vi "Alarms Wizard.vi"(8 "error in":errorcluster, 11 "Shared Variable Name":string) -> (0 "error out":errorcluster, 2 "Cancel":bool, 3 "alarm settings":T1={"enable? (F)"=FALSE, "name"="HiHi", "alarm type"=enum."HI_HI", "level/change"=90.0, "deadband/time"=1.0, "priority"=1, "ack type"=enum."Auto", "area"="", "description"="", "log? (T)"=TRUE} {"priority" min=1 max=5000})   [LabVIEW 2020]
uses:
  <vilib>/lvdsc/variables/internal/AlarmSettings_Numeric.ctl
  <vilib>/lvdsc/variables/internal/NumericAlarmType.ctl
panel:
  in  "OK Button":bool
  in  "Cancel Button":bool
  in  "Next Button":bool
  in  "Previous Button":bool
  in  "Tab Control":enum32{"1", "2", "3", "4", "5", "6", "7"}(tab)
  in  "alarm type":enum16{"HI_HI", "HI", "LO", "LO_LO"}(ring)
  in  "Set Point":dbl
  in  "deadband":dbl
  in  "priority":enum16{"Low", "Moderate", "High", "Critical"}(ring)
  in  "area":string
  in  "description":string
  in  "log?":bool
  # "Select the Alarm Type"
  # "Users may configure upto 4 alarms for each\nvariable. \nHI_HI and HI are High level Alarms\ntriggered when varaible value goes over the\nsetpoint. \nLO_LO and LO are Low level alarms\nthat are triggered when variable value falls\nbelow the setpoint."
  # "Enter the Set Point"
  # "A setpoint is the threshold for the alarm. The \nalarm is trigger when variable value crosses\nthis threshold."
  # "Enter the deadband"
  # "Deadband is range of values above or below \nthe alarm threshold. It prevents frequent\ntoggling of alarms if the variable value is \nnoisy around the threshold value.\n\nFor example, if the Setpoint for a HI alarm is \n1200 and the deadband is 50, the alarm will be \ntriggered when the variable value is greater\nthan 1200 and will remain Active until it falls\nbelow 1150."
  # "Set the Priority Level"
  # "The Priority Level allows the user to set up \nthe severity of the alarm. There are 4 levels\navailable. User alerts for alarms vary based on\nthe priority level set for the alarm."
  # "Enter Area/Location"
  # "Provide the name of the Area for which the \nvaraible is being logged and monitored\nfor alarms."
  # "Enter Description"
  # "Provide a description for the Alarm. \nFor example, \" Hi Alarm for Cryo1 Temp\""
  # "Do you want to Log this Alarm?"
  # "Click on this button to toggle between choices.\nUsers may choose to log this alarm event\nin a database. This will provide a history for\nthis alarm."
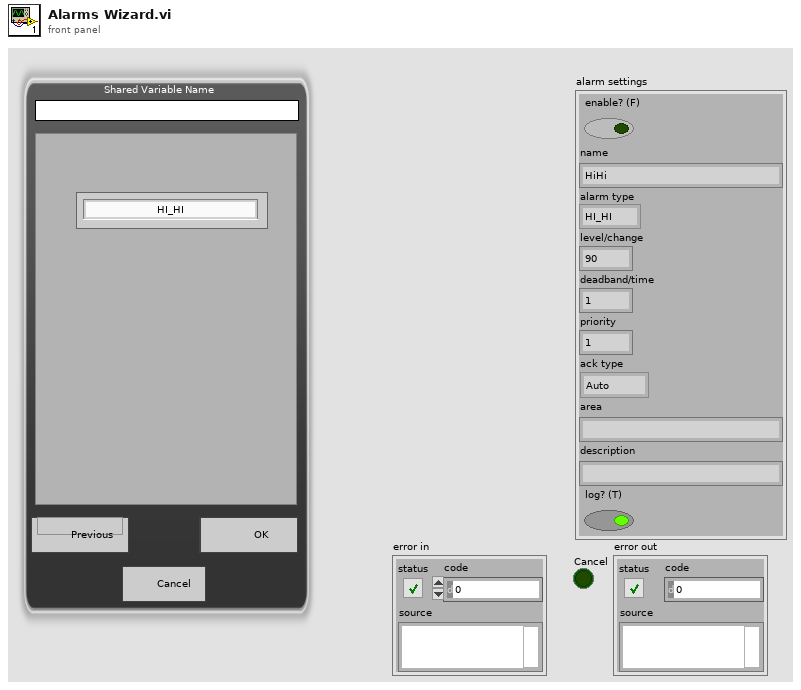
[diagram p1: front panel]
types:
  T1 = typedef "AlarmSettings_Numeric.ctl" = cluster{"enable? (F)":bool, "name":string, "alarm type":T2, "level/change":dbl, "deadband/time":dbl, "priority":u32, "ack type":enum16{"Auto", "User", "None", "Each Occurrence"}, "area":string, "description":string, "log? (T)":bool}
  T2 = typedef "NumericAlarmType.ctl" = enum16{"HI_HI", "HI", "LO", "LO_LO"}
  T3 = enum32{"invalid app kind", "Development System", "Run Time System", "Student Edition", "Embedded LabVIEW", "Evaluation", "Custom"}
  T4 = enum32{"Invalid", "Standard", "Closed", "Hidden", "Minimized", "Maximized"}
  T5 = cluster{"Core":cluster{"Current VI Reference":refnum<vi>, "Close Panel on Exit?":bool}, "No of pages":i32, "alarm settings":T1}
  T6 = cluster{"Current VI Reference":refnum<vi>, "Close Panel on Exit?":bool}
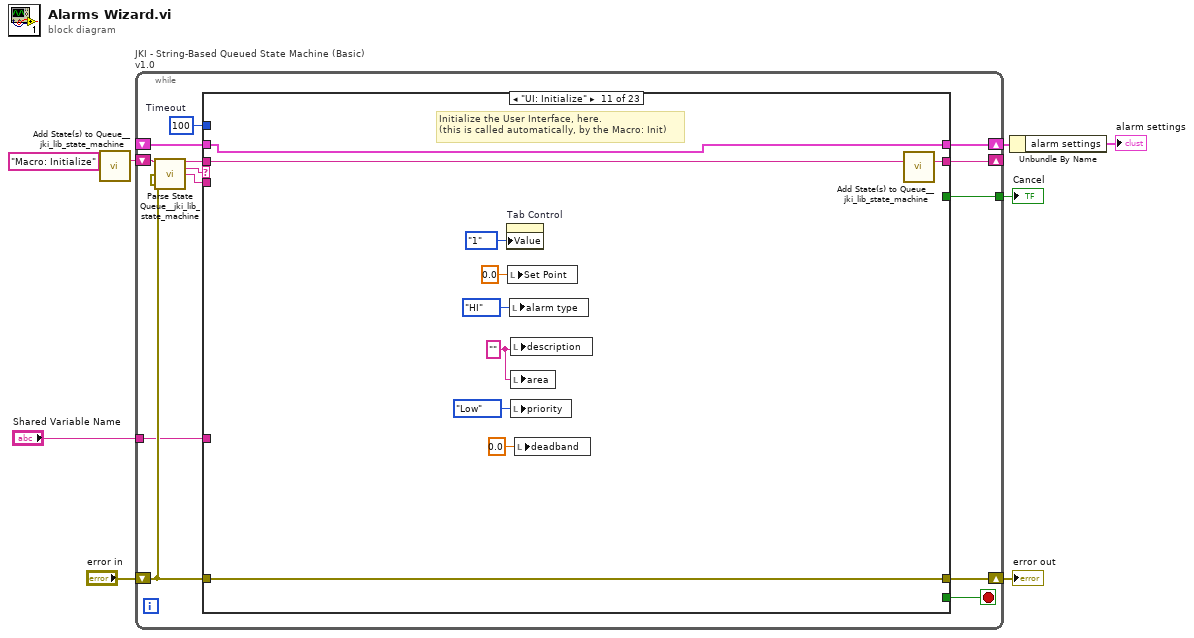
[diagram p0: block diagram]
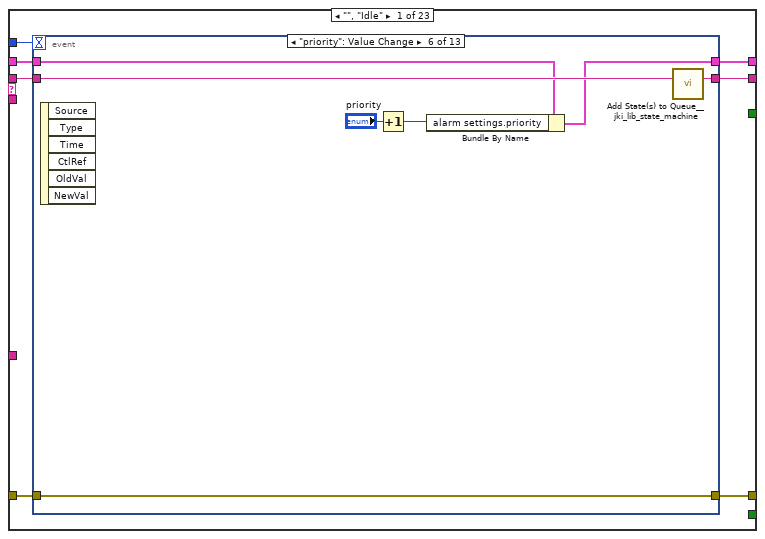
[diagram p2: hidden frame]
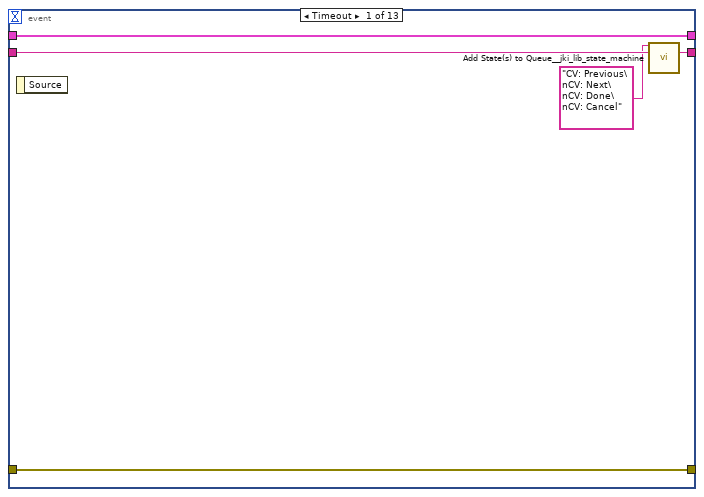
[diagram p3: hidden frame]
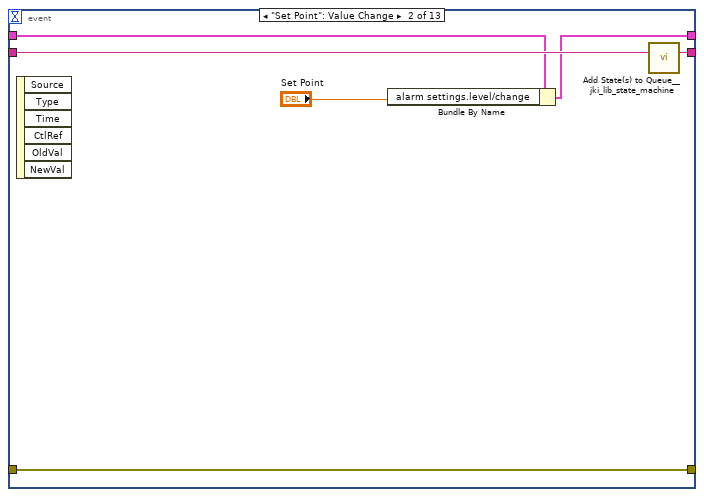
[diagram p4: hidden frame]
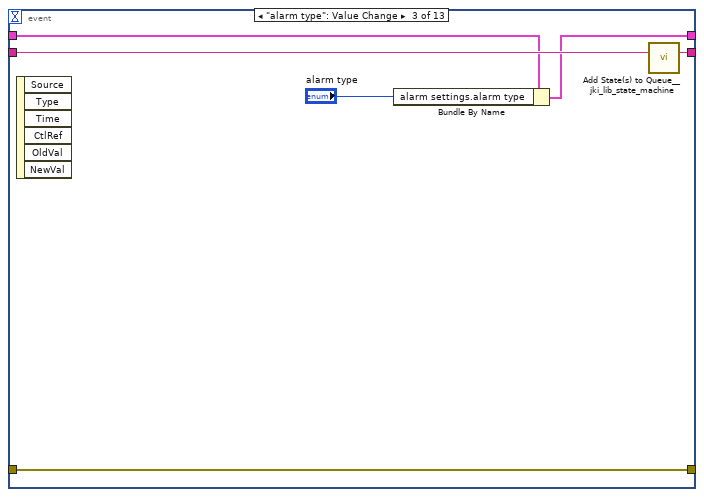
[diagram p5: hidden frame]
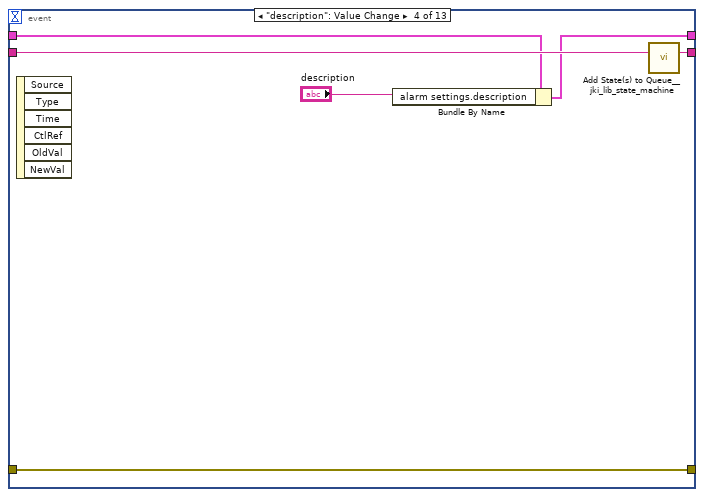
[diagram p6: hidden frame]
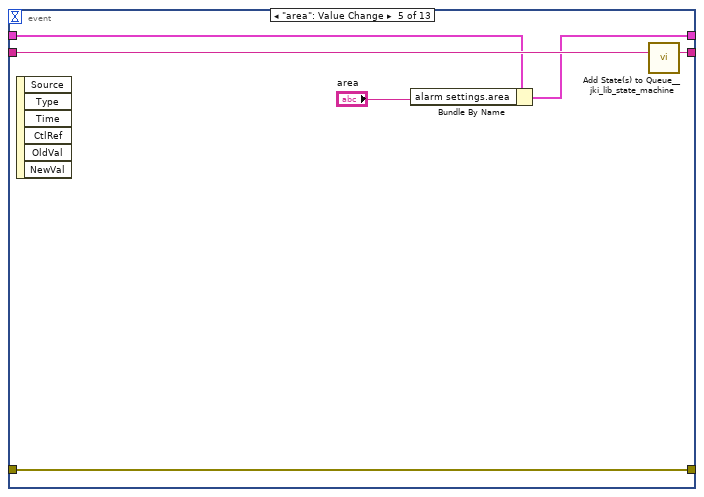
[diagram p7: hidden frame]
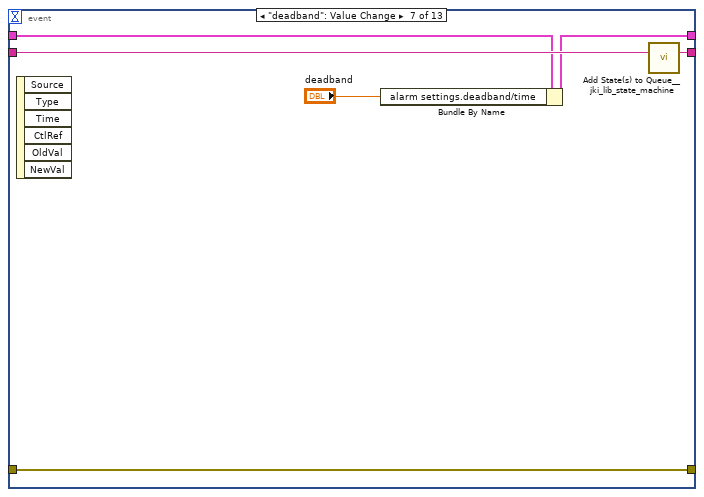
[diagram p8: hidden frame]
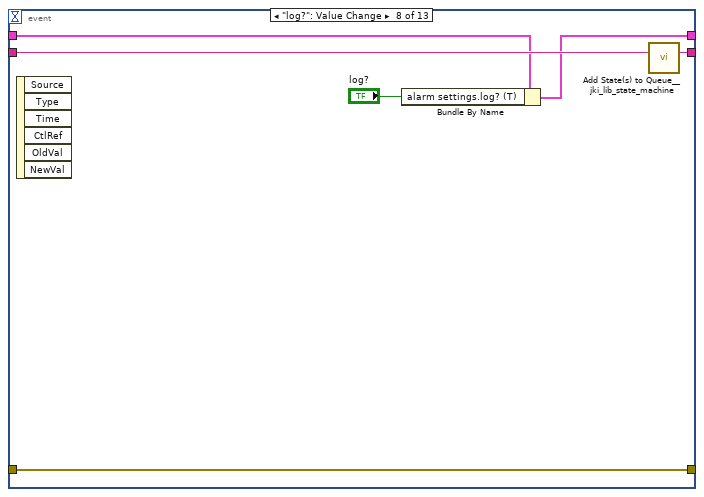
[diagram p9: hidden frame]
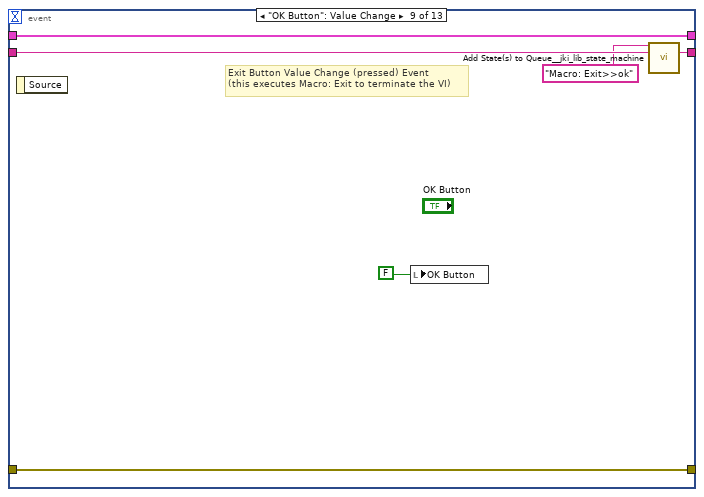
[diagram p10: hidden frame]
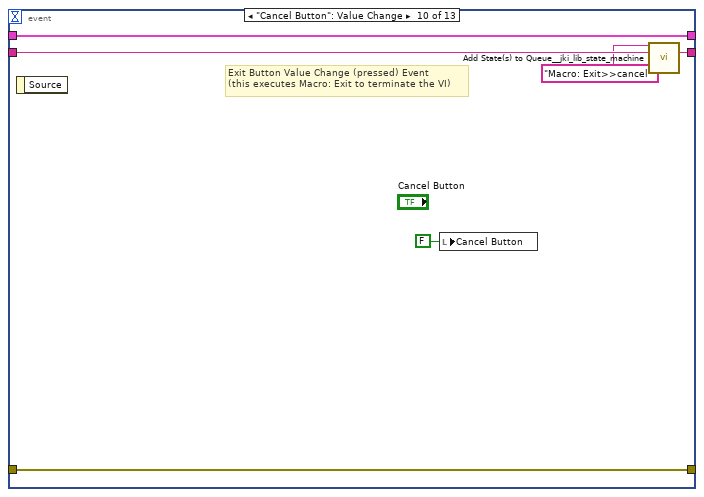
[diagram p11: hidden frame]
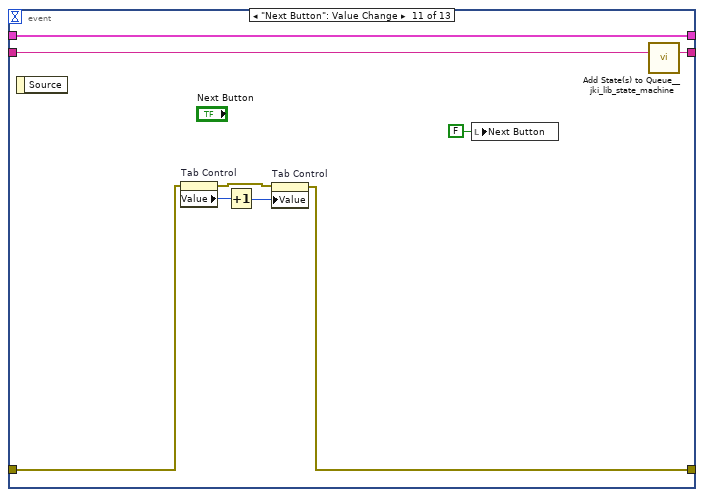
[diagram p12: hidden frame]
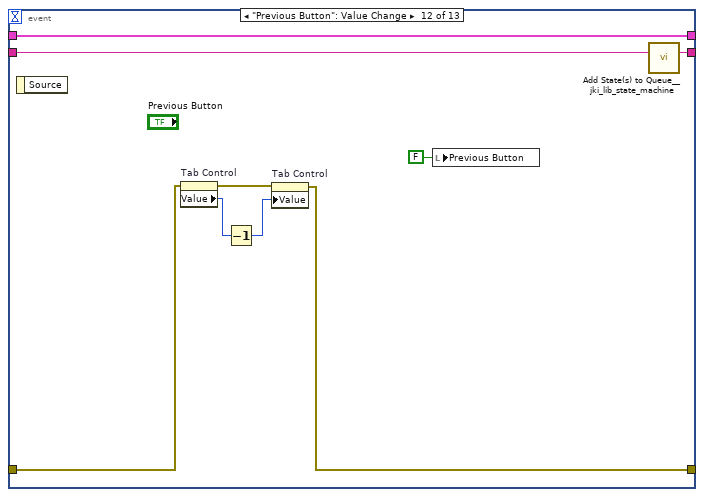
[diagram p13: hidden frame]
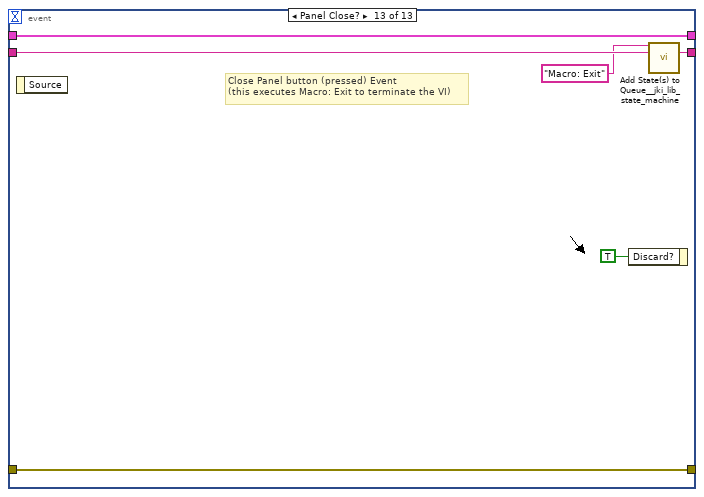
[diagram p14: hidden frame]
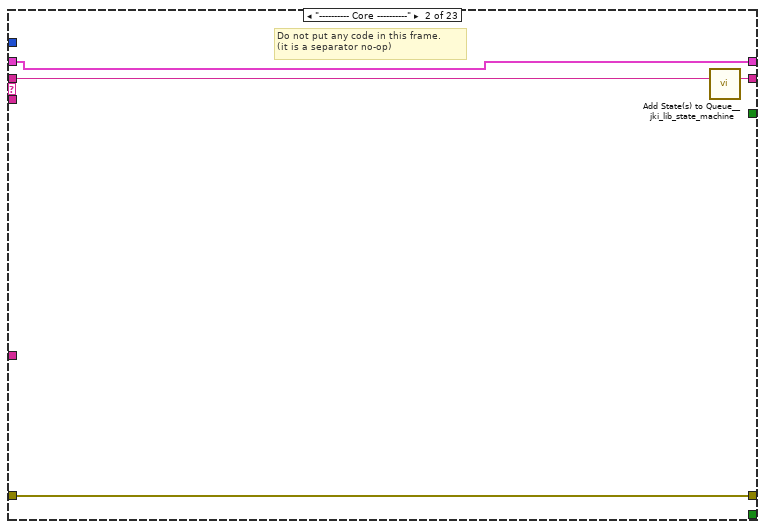
[diagram p15: hidden frame]
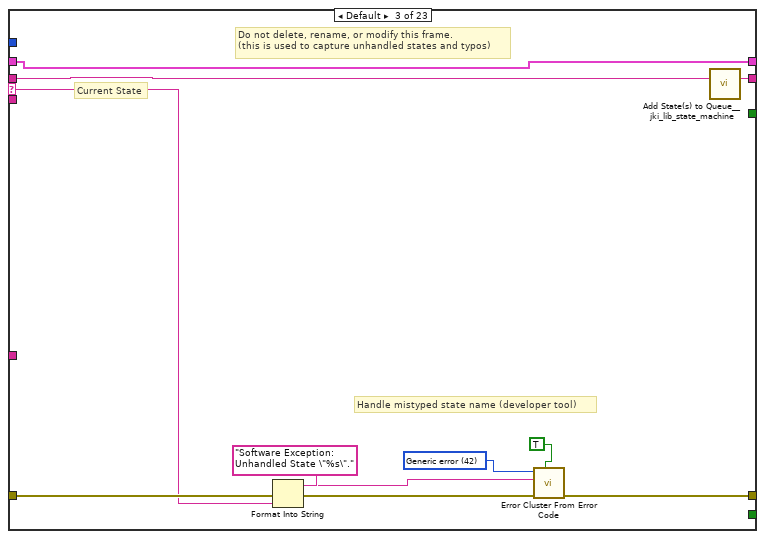
[diagram p16: hidden frame]
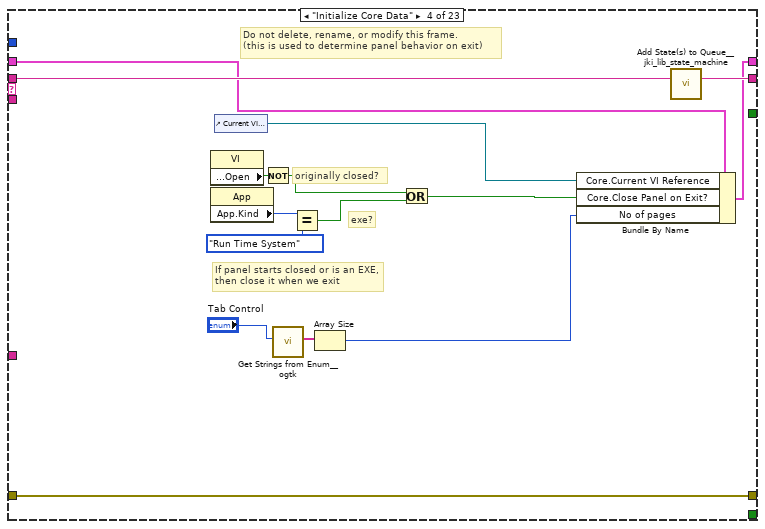
[diagram p17: hidden frame]
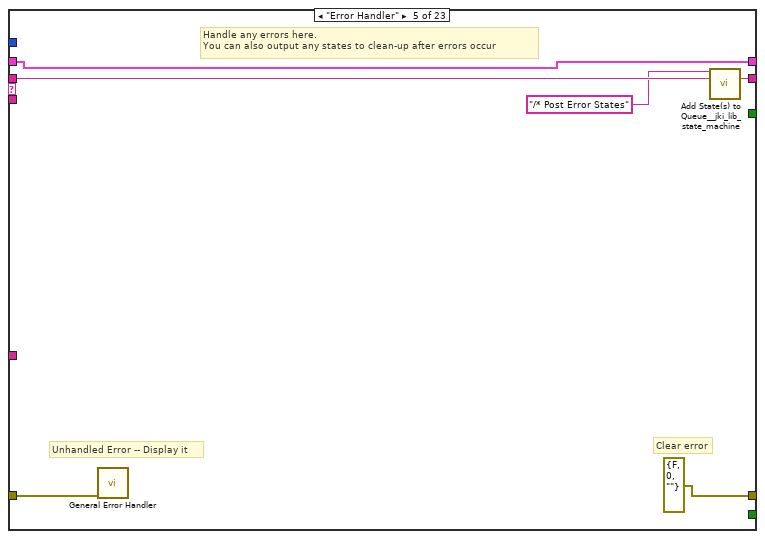
[diagram p18: hidden frame]
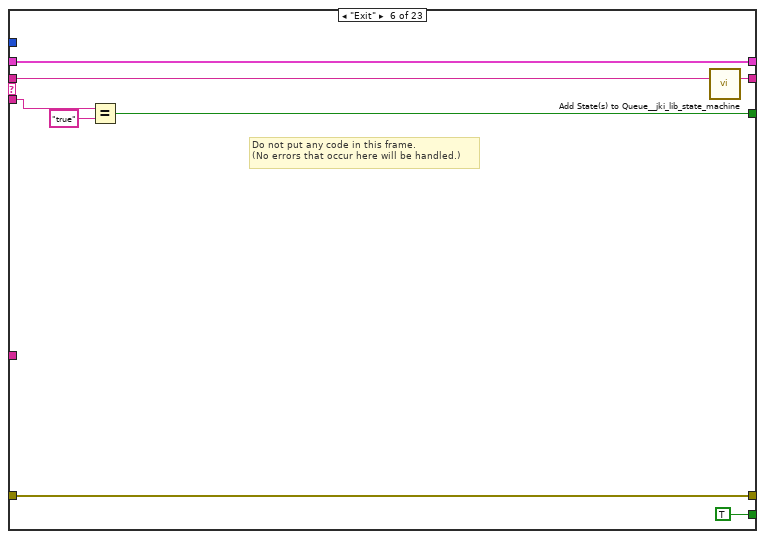
[diagram p19: hidden frame]
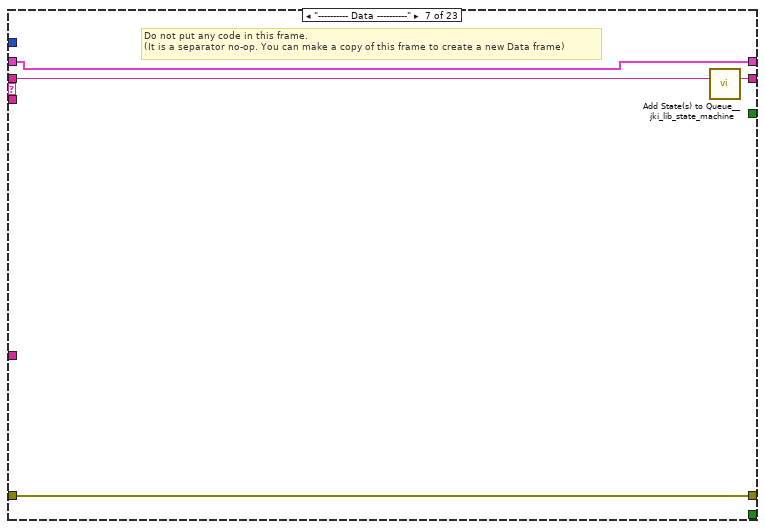
[diagram p20: hidden frame]
diagram:
  n1 = call <vilib>:"Add State(s) to Queue__jki_lib_state_machine.vi"("State(s) in (\"\")"="Macro: Initialize") -> ("States Out"=w8:string)  [unwired: 14 in]
  n2 = while "JKI - String-Based Queued State Machine (Basic) v1.0" {
    shift-right: [w14] -> w4
    shift-left: _ -> [w13]
    shift-right: [w17] -> w1
    shift-left: "error in" -> [w11]
    shift-right: [w16] -> _
    shift-left: w8 -> [w18]
    tunnel: "Shared Variable Name" -> [w10]
    tunnel: [w9] -> w5
    stop <- w15 stop-if-true
    w12 = 100  # Timeout
    n3 = call <vilib>:"Parse State Queue__jki_lib_state_machine.vi"("State Queue"=w18, "Error In (no error)"=w11) -> ("Remaining States"=w20:string, "Current State"=w21:string, "Arguments"=w19:string)  [unwired: 11 in]
    n4 = case shown="\"UI: Initialize\"" w21 {
      selector: w21 -> [_ _ w117 _ _ _ _ _ _ _ _ _ _ _ _ _ _ _ _ _ _ _ _]
      tunnel: w20 -> [w28 w116 w121 w142 w148 w156 w160 w169 w175 w179 w189 w195 w206 w232 w237 w252 w256 w265 w276 w286 w290 w294 w298]
      tunnel: w19 -> [_ _ _ _ _ w151 _ _ _ _ _ w190 w200 _ _ w243 _ _ _ _ _ _ _]
      tunnel: w13 -> [w26 w113 w119 w133 w145 w154 w157 _ w170 w176 w187 w193 w202 w229 w234 w249 w253 w262 w273 w283 w287 w291 w295]
      tunnel: [w25 w114 w123 w139 errorcluster {"status"=FALSE, "code"=0, "source"=""} ("error out") w153 w158 w166 w171 w177 w186 w191 w203 w230 w235 w250 w254 w257 w274 w284 w288 w292 w296] -> w17
      tunnel: w11 -> [w24 w114 w122 w139 w144 w153 w158 w166 w172 w177 w186 w192 w204 w230 w235 w250 w254 w258 w274 w284 w288 w292 w296]
      tunnel: [w27 w115 w120 w141 w147 w155 w159 w168 w174 w178 w188 w194 w205 w231 w236 w251 w255 w264 w275 w285 w289 w293 w297] -> w16
      tunnel: [_ _ _ _ _ TRUE _ _ _ _ _ _ _ _ _ _ _ _ _ _ _ _ _] -> w15
      tunnel: [w23 w113 w119 w140 w145 w154 w157 w167 w170 w176 w187 w193 w202 w229 w234 w249 w253 w262 w273 w283 w287 w291 w295] -> w14
      tunnel: w12 -> [w22 _ _ _ _ _ _ _ _ _ _ _ _ _ _ _ _ _ _ _ _ _ _]
      tunnel: w10 -> [_ _ _ _ _ _ _ w162 _ _ _ _ _ _ _ _ _ _ _ _ _ _ _]
      tunnel: [_ _ _ _ _ w149 _ _ _ _ _ _ _ _ _ _ _ _ _ _ _ _ _] -> w9
      frame "", "Idle" {
        n5 = event shown="[5] \"priority\": Value Change" {
          selector: _ -> [_ _ _ _ _ _ _ _ _ _ _ _ _]
          dyn-events: _ -> [_ _ _ _ _ _ _ _ _ _ _ _ _]
          timeout: w22 -> [_ _ _ _ _ _ _ _ _ _ _ _ _]
          tunnel: w28 -> [w33 w39 w45 w51 w57 w64 w70 w76 w82 w88 w97 w106 w112]
          tunnel: [w32 w38 w44 w50 w56 w63 w69 w75 w81 w87 w96 w105 w111] -> w27
          tunnel: w26 -> [w30 w36 w42 w48 w54 w61 w67 w73 w79 w85 w95 w104 w109]
          tunnel: [w31 w37 w43 w49 w55 w62 w68 w74 w80 w86 w90 w99 w110] -> w25
          tunnel: w24 -> [w31 w37 w43 w49 w55 w62 w68 w74 w80 w86 w91 w100 w110]
          tunnel: [w30 w35 w41 w47 w53 w60 w66 w72 w79 w85 w95 w104 w109] -> w23
          event Timeout {
            n6 = event-data() -> ()  [unwired: 1 in, 1 out]
            n7 = call <vilib>:"Add State(s) to Queue__jki_lib_state_machine.vi"("State(s) in Front (\"\")"="CV: Previous\nCV: Next\nCV: Done\nCV: Cancel", "State(s) in (\"\")"=w33) -> ("States Out"=w32:string)  [unwired: 13 in]
          }
          event "Set Point": Value Change {
            n8 = event-data() -> ()  [unwired: 1 in, 6 out]
            n9 = Bundle By Name(cluster=w36, "alarm settings.level/change"="Set Point") -> (w35:T5)
            n10 = call <vilib>:"Add State(s) to Queue__jki_lib_state_machine.vi"("State(s) in (\"\")"=w39) -> ("States Out"=w38:string)  [unwired: 14 in]
          }
          event "alarm type": Value Change {
            n11 = event-data() -> ()  [unwired: 1 in, 6 out]
            n12 = Bundle By Name(cluster=w42, "alarm settings.alarm type"="alarm type") -> (w41:T5)
            n13 = call <vilib>:"Add State(s) to Queue__jki_lib_state_machine.vi"("State(s) in (\"\")"=w45) -> ("States Out"=w44:string)  [unwired: 14 in]
          }
          event "description": Value Change {
            n14 = event-data() -> ()  [unwired: 1 in, 6 out]
            n15 = Bundle By Name(cluster=w48, "alarm settings.description"="description") -> (w47:T5)
            n16 = call <vilib>:"Add State(s) to Queue__jki_lib_state_machine.vi"("State(s) in (\"\")"=w51) -> ("States Out"=w50:string)  [unwired: 14 in]
          }
          event "area": Value Change {
            n17 = event-data() -> ()  [unwired: 1 in, 6 out]
            n18 = Bundle By Name(cluster=w54, "alarm settings.area"="area") -> (w53:T5)
            n19 = call <vilib>:"Add State(s) to Queue__jki_lib_state_machine.vi"("State(s) in (\"\")"=w57) -> ("States Out"=w56:string)  [unwired: 14 in]
          }
          event "priority": Value Change {
            n20 = event-data() -> ()  [unwired: 1 in, 6 out]
            n21 = Increment(x="priority") -> (x+1=w58:enum16{"Low", "Moderate", "High", "Critical"})
            n22 = Bundle By Name(cluster=w61, "alarm settings.priority"=w58) -> (w60:T5)
            n23 = call <vilib>:"Add State(s) to Queue__jki_lib_state_machine.vi"("State(s) in (\"\")"=w64) -> ("States Out"=w63:string)  [unwired: 14 in]
          }
          event "deadband": Value Change {
            n24 = event-data() -> ()  [unwired: 1 in, 6 out]
            n25 = Bundle By Name(cluster=w67, "alarm settings.deadband/time"="deadband") -> (w66:T5)
            n26 = call <vilib>:"Add State(s) to Queue__jki_lib_state_machine.vi"("State(s) in (\"\")"=w70) -> ("States Out"=w69:string)  [unwired: 14 in]
          }
          event "log?": Value Change {
            n27 = event-data() -> ()  [unwired: 1 in, 6 out]
            n28 = Bundle By Name(cluster=w73, "alarm settings.log? (T)"="log?") -> (w72:T5)
            n29 = call <vilib>:"Add State(s) to Queue__jki_lib_state_machine.vi"("State(s) in (\"\")"=w76) -> ("States Out"=w75:string)  [unwired: 14 in]
          }
          event "OK Button": Value Change {
            # "Exit Button Value Change (pressed) Event\n(this executes Macro: Exit to terminate the VI)"
            n30 = event-data() -> ()  [unwired: 1 in, 1 out]
            n31 = local write "OK Button"(FALSE ("OK Button")) -> ()
            n32 = call <vilib>:"Add State(s) to Queue__jki_lib_state_machine.vi"("State(s) in Front (\"\")"="Macro: Exit>>ok", "State(s) in (\"\")"=w82) -> ("States Out"=w81:string)  [unwired: 13 in]
          }
          event "Cancel Button": Value Change {
            # "Exit Button Value Change (pressed) Event\n(this executes Macro: Exit to terminate the VI)"
            n33 = event-data() -> ()  [unwired: 1 in, 1 out]
            n34 = local write "Cancel Button"(FALSE ("Cancel Button")) -> ()
            n35 = call <vilib>:"Add State(s) to Queue__jki_lib_state_machine.vi"("State(s) in Front (\"\")"="Macro: Exit>>cancel", "State(s) in (\"\")"=w88) -> ("States Out"=w87:string)  [unwired: 13 in]
          }
          event "Next Button": Value Change {
            n36 = event-data() -> ()  [unwired: 1 in, 1 out]
            n37 = property on="Tab Control" class="TabCtl (strict)"(error in=w91) -> (error out=w92:errorcluster, "Value"=w94:enum32{"1", "2", "3", "4", "5", "6", "7"})  [unwired: 1 in, 1 out]
            n38 = Increment(x=w94) -> (x+1=w93:enum32{"1", "2", "3", "4", "5", "6", "7"})
            n39 = property on="Tab Control" class="TabCtl (strict)"(error in=w92, "Value"=w93) -> (error out=w90:errorcluster)  [unwired: 1 in, 1 out]
            n40 = local write "Next Button"(FALSE ("Next Button")) -> ()
            n41 = call <vilib>:"Add State(s) to Queue__jki_lib_state_machine.vi"("State(s) in (\"\")"=w97) -> ("States Out"=w96:string)  [unwired: 14 in]
          }
          event "Previous Button": Value Change {
            n42 = event-data() -> ()  [unwired: 1 in, 1 out]
            n43 = property on="Tab Control" class="TabCtl (strict)"(error in=w100) -> (error out=w101:errorcluster, "Value"=w103:enum32{"1", "2", "3", "4", "5", "6", "7"})  [unwired: 1 in, 1 out]
            n44 = Decrement(x=w103) -> (x-1=w102:enum32{"1", "2", "3", "4", "5", "6", "7"})
            n45 = property on="Tab Control" class="TabCtl (strict)"(error in=w101, "Value"=w102) -> (error out=w99:errorcluster)  [unwired: 1 in, 1 out]
            n46 = local write "Previous Button"(FALSE ("Previous Button")) -> ()
            n47 = call <vilib>:"Add State(s) to Queue__jki_lib_state_machine.vi"("State(s) in (\"\")"=w106) -> ("States Out"=w105:string)  [unwired: 14 in]
          }
          event Panel Close? {
            # "Close Panel button (pressed) Event\n(this executes Macro: Exit to terminate the VI)"
            n48 = event-data() -> ()  [unwired: 1 in, 1 out]
            n49 = event-data("Discard?"=TRUE) -> ()  [unwired: 1 in, 1 out]
            n50 = call <vilib>:"Add State(s) to Queue__jki_lib_state_machine.vi"("State(s) in Front (\"\")"="Macro: Exit", "State(s) in (\"\")"=w112) -> ("States Out"=w111:string)  [unwired: 13 in]
          }
        }
      }
      frame "---------- Core ----------" {
        # "Do not put any code in this frame.\n(it is a separator no-op)"
        n51 = call <vilib>:"Add State(s) to Queue__jki_lib_state_machine.vi"("State(s) in (\"\")"=w116) -> ("States Out"=w115:string)  [unwired: 14 in]
      }
      frame Default {
        w126 = 42 items=["No error", "Argument error", "Memory is full", "Out of zone", "End of file", "File already open", "Generic file I/O error", "File not found", "File permission error", "Disk is full", "Duplicate path", "Too many files open", "System feature not enabled", "Resource file not found", "Cannot add resource", "Resource not found", "Image not found", "Image memory error", "Pen does not exist", "Config type invalid", "Config token not found", "Config parse error", "Config memory error", "Bad external code format", "Bad external code offset", "External code not present", "Null window", "Destroy window error", "Null menu", "Print aborted", "Bad print record", "Print driver error", "Windows error during printing", "Memory error during printing", "Print dialog error", "Generic print error", "Invalid device refnum", "Device not found", "Device parameter error", "Device unit error", "Cannot open device", "Device call aborted", "Generic error", "Cancelled by user", "Object ID too low", "Object ID too high", "Object not in heap", "Unknown heap", "Unknown object (invalid DefProc)", "Unknown object (DefProc not in table)", "Message out of range", "Invalid (null) method", "Unknown message", "Manager call not supported", "Bad address", "Network operation in progress", "Network operation timed out", "Connection is busy", "Network attribute not supported", "Network error", "Address in use", "System out of memory", "Connection aborted", "Connection refused", "Not connected", "Already connected", "Connection closed", "Initialization error (interapplication manager)", "Bad occurrence", "Wait on unbound occurrence handler", "Occurrence queue overflow", "Datalog type conflict", "Unused", "Unrecognized type (interapplication manager)", "Memory corrupt", "Failed to make temporary DLL", "Old CIN version", "Drag socket not found", "Failed to load drop-object", "Failed to register OLE object", "Failed to release OLE object", "Format specifier type mismatch", "Unknown format specifier", "Too few format specifiers", "Too many format specifiers", "Scan failed", "Newer CIN version", "Error converting to variant", "Runtime menu error", "Password tampered", "Variant attribute not found", "Incompatible variant data type", "Event data is not available", "Event Store is not present", "Occurrence is not found", "Event Queue is not created", "Event info is not available", "Refnum passed is NULL", "Error retrieving Class GUID", "Error retrieving CoClass GUID", "Error retrieving TypeLib GUID.", "Bad built application magic bytes.", "Specific driver is different from the specific driver associated with the Logical Name.", "There is no session opened to the class driver.", "Max Error", "MAX - Error with config objects", "MAX - Error loading configuration", "MAX - Group not supported"]
        # "Current State"
        # "Do not delete, rename, or modify this frame.\n(this is used to capture unhandled states and typos)"
        # "Handle mistyped state name (developer tool)"
        n52 = Format Into String(format string="Software Exception: Unhandled State \"%s\"." ("message"), error in=w122, w117) -> (resulting string=w125:string, error out=w124:errorcluster)  [unwired: 1 in]
        n53 = call <vilib>:"Error Cluster From Error Code.vi"("show call chain? (False)"=TRUE, "error in (no error)"=w124, "error message (\"\")"=w125, "error code (0)"=w126) -> ("error out"=w123:errorcluster)  [unwired: 5 in]
        n54 = call <vilib>:"Add State(s) to Queue__jki_lib_state_machine.vi"("State(s) in (\"\")"=w121) -> ("States Out"=w120:string)  [unwired: 14 in]
      }
      frame "Initialize Core Data" {
        # "Do not delete, rename, or modify this frame.\n(this is used to determine panel behavior on exit)"
        # "originally closed?"
        # "exe?"
        # "If panel starts closed or is an EXE, then close it when we exit"
        n55 = property class="VI"() -> ("Front Panel.Open"=w138:bool)  [unwired: 2 in, 2 out]
        n56 = property class="App"() -> ("App.Kind"=w137:T3)  [unwired: 2 in, 2 out]
        n57 = control-ref of="Current VI Reference"() -> (w131:refnum<vi>)
        n58 = Not(x=w138) -> (.not. x?=w135:bool)
        n59 = call <userlib>:"Get Strings from Enum__ogtk.vi"("Enum"="Tab Control") -> ("Enum Strings"=w130:string[])  [unwired: 7 in, 3 out]
        n60 = Equal?(x=w137, y=T3."Run Time System" ("Application:Kind")) -> (x = y?=w134:bool)
        n61 = Array Size(array=w130) -> (size(s)=w128:i32)
        n62 = Or(x=w135, y=w134) -> (x .or. y?=w132:bool)
        n63 = Bundle By Name(cluster=w133, "Core.Current VI Reference"=w131, "Core.Close Panel on Exit?"=w132, "No of pages"=w128) -> (w140:T5)
        n64 = call <vilib>:"Add State(s) to Queue__jki_lib_state_machine.vi"("State(s) in (\"\")"=w142) -> ("States Out"=w141:string)  [unwired: 14 in]
      }
      frame "Error Handler" {
        # "Unhandled Error -- Display it"
        # "Handle any errors here.\nYou can also output any states to clean-up after errors occur"
        # "Clear error"
        n65 = call <vilib>:"General Error Handler.vi"("error in (no error)"=w144) -> ()  [unwired: 10 in, 5 out]
        n66 = call <vilib>:"Add State(s) to Queue__jki_lib_state_machine.vi"("State(s) in Front (\"\")"="/* Post Error States", "State(s) in (\"\")"=w148) -> ("States Out"=w147:string)  [unwired: 13 in]
      }
      frame "Exit" {
        # "Do not put any code in this frame.\n(No errors that occur here will be handled.)"
        n67 = Equal?(x=w151, y="true") -> (x = y?=w149:bool)
        n68 = call <vilib>:"Add State(s) to Queue__jki_lib_state_machine.vi"("State(s) in (\"\")"=w156) -> ("States Out"=w155:string)  [unwired: 14 in]
      }
      frame "---------- Data ----------" {
        # "Do not put any code in this frame.\n(It is a separator no-op. You can make a copy of this frame to create a new Data frame)"
        n69 = call <vilib>:"Add State(s) to Queue__jki_lib_state_machine.vi"("State(s) in (\"\")"=w160) -> ("States Out"=w159:string)  [unwired: 14 in]
      }
      frame "Data: Initialize" {
        w163 = T1 {"enable? (F)"=TRUE, "name"="", "alarm type"=enum."HI", "level/change"=0.0, "deadband/time"=0.0, "priority"=1, "ack type"=enum."Auto", "area"="", "description"="", "log? (T)"=FALSE}  # alarm settings
        w164 = 0  # No of pages
        w165 = T6 {"Current VI Reference"=refnum, "Close Panel on Exit?"=FALSE}  # Core
        # "Initialize the shift-register data, here.\n(data names are defined by what you wire into the bundle function)"
        n70 = Bundle By Name(cluster=w163, "name"=w162) -> (w161:T1)
        n71 = Bundle("Core"=w165, "No of pages"=w164, "alarm settings"=w161) -> (w167:T5)  [unwired: 1 in]
        n72 = call <vilib>:"Add State(s) to Queue__jki_lib_state_machine.vi"("State(s) in (\"\")"=w169) -> ("States Out"=w168:string)  [unwired: 14 in]
      }
      frame "Data: Cleanup" {
        # "Cleanup any data and references, here.\n(this is called automatically, by the Macro: Exit)"
        n73 = Unbundle By Name(w170) -> ("Core.Current VI Reference"=w173:refnum<vi>)
        n74 = Close Reference(reference=w173, error in (no error)=w172) -> (error out=w171:errorcluster)
        n75 = call <vilib>:"Add State(s) to Queue__jki_lib_state_machine.vi"("State(s) in (\"\")"=w175) -> ("States Out"=w174:string)  [unwired: 14 in]
      }
      frame "---------- UI ----------" {
        # "Do not put any code in this frame.\n(It is a separator no-op. You can make a copy of this frame to create a new UI frame)"
        n76 = call <vilib>:"Add State(s) to Queue__jki_lib_state_machine.vi"("State(s) in (\"\")"=w179) -> ("States Out"=w178:string)  [unwired: 14 in]
      }
      frame "UI: Initialize" {
        w183 = "" ("description")
        # "Initialize the User Interface, here.\n(this is called automatically, by the Macro: Init)"
        n77 = property on="Tab Control" class="TabCtl (strict)"("Value"=enum32{"1", "2", "3", "4", "5", "6", "7"}."1" ("Tab Control")) -> ()  [unwired: 2 in, 2 out]
        n78 = local write "Set Point"(0.0 ("Set Point")) -> ()
        n79 = local write "alarm type"(enum16{"HI_HI", "HI", "LO", "LO_LO"}."HI" ("alarm type")) -> ()
        n80 = local write "description"(w183) -> ()
        n81 = local write "area"(w183) -> ()
        n82 = local write "priority"(enum16{"Low", "Moderate", "High", "Critical"}."Low" ("priority")) -> ()
        n83 = local write "deadband"(0.0 ("deadband")) -> ()
        n84 = call <vilib>:"Add State(s) to Queue__jki_lib_state_machine.vi"("State(s) in (\"\")"=w189) -> ("States Out"=w188:string)  [unwired: 14 in]
      }
      frame "UI: Cursor Set" {
        # "Argument"
        # "Set and Unset Cursor Busy.\n(Usage: \"UI: Cursor Set >> Busy|Idle\")"
        n85 = case shown="\"Idle\", Default" w190 {
          tunnel: w192 -> [w197 w199]
          tunnel: [w196 w198] -> w191
          frame "Idle", Default {
            n86 = call <vilib>:"Unset Busy.vi"("error in (no error)"=w197) -> ("error out"=w196:errorcluster)  [unwired: 10 in]
          }
          frame "Busy" {
            n87 = call <vilib>:"Set Busy.vi"("error in (no error)"=w199) -> ("error out"=w198:errorcluster)  [unwired: 9 in, 1 out]
          }
        }
        n88 = call <vilib>:"Add State(s) to Queue__jki_lib_state_machine.vi"("State(s) in (\"\")"=w195) -> ("States Out"=w194:string)  [unwired: 14 in]
      }
      frame "UI: Front Panel State" {
        # "Argument"
        # "Set Front Panel Open or Closed\n(Usage: \"UI: Front Panel State >> Open|Close\")"
        n89 = Unbundle By Name(w202) -> ("Core.Current VI Reference"=w201:refnum<vi>)
        n90 = case shown="\"Open\", Default" w200 {
          tunnel: w204 -> [w210 w223]
          tunnel: [w212 w224] -> w203
          tunnel: w201 -> [w211 w221]
          frame "Open", Default {
            n91 = property class="VI"(reference=w211, error in=w210) -> (reference out=w208:refnum<vi>, error out=w209:errorcluster, "Front Panel.Open"=w207:bool)
            n92 = case shown="False" w207 {
              tunnel: [w215 w218] -> w212
              tunnel: w209 -> [w214 w218]
              tunnel: w208 -> [w213 _]
              frame False {
                n93 = invoke class="VI" method="FP.Open"(reference=w213, error in=w214, "Activate"=TRUE, "State"=T4."Standard") -> (error out=w215:errorcluster)  [unwired: 1 in, 4 out]
              }
              frame True {
              }
            }
          }
          frame "Close" {
            n94 = property class="VI"(reference=w221, error in=w223) -> (reference out=w220:refnum<vi>, error out=w222:errorcluster, "Front Panel.Open"=w219:bool)
            n95 = case shown="True" w219 {
              tunnel: [w225 w228] -> w224
              tunnel: w222 -> [w225 w227]
              tunnel: w220 -> [_ w226]
              frame False {
              }
              frame True {
                n96 = invoke class="VI" method="FP.Close"(reference=w226, error in=w227) -> (error out=w228:errorcluster)  [unwired: 1 in, 2 out]
              }
            }
          }
        }
        n97 = call <vilib>:"Add State(s) to Queue__jki_lib_state_machine.vi"("State(s) in (\"\")"=w206) -> ("States Out"=w205:string)  [unwired: 14 in]
      }
      frame "---------- Macro ----------" {
        # "Do not put any code in this frame.\n(It is a separator no-op. You can make a copy of this frame to create a new Macro frame)"
        n98 = call <vilib>:"Add State(s) to Queue__jki_lib_state_machine.vi"("State(s) in (\"\")"=w232) -> ("States Out"=w231:string)  [unwired: 14 in]
      }
      frame "Macro: Initialize" {
        w233 = "Data: Initialize\nInitialize Core Data\nUI: Initialize\nUI: Front Panel State >> Open"  # Data: Initialize Initialize Core Data UI: Initialize UI: Front Panel State >> Open
        # "Initialization Macro\n(This is called once, when the VI starts)"
        n99 = call <vilib>:"Add State(s) to Queue__jki_lib_state_machine.vi"("State(s) in Front (\"\")"=w233, "State(s) in (\"\")"=w237) -> ("States Out"=w236:string)  [unwired: 13 in]
      }
      frame "Macro: Exit" {
        # "Exit Macro\n(This is called once, when the VI exits)"
        n100 = Unbundle By Name(w249) -> ("Core.Close Panel on Exit?"=w248:bool)
        n101 = Equal?(x=w243, y="cancel") -> (x = y?=w241:bool)
        n102 = Select(t="Data: Cleanup\nExit>>true", s=w241, f="Data: Cleanup\nExit>>false") -> (s? t:f=w238:string)
        n103 = Select(t="UI: Front Panel State >> Close", s=w248, f="") -> (s? t:f=w245:string)
        n104 = call <vilib>:"Add State(s) to Queue__jki_lib_state_machine.vi"("State(s) in (\"\")"=w245, "State(s) at Back (\"\")"=w238) -> ("States Out"=w244:string)  [unwired: 13 in]
        n105 = call <vilib>:"Add State(s) to Queue__jki_lib_state_machine.vi"("State(s) in Front (\"\")"=w244, "State(s) in (\"\")"=w252) -> ("States Out"=w251:string)  [unwired: 13 in]
      }
      frame "---------- ControlsVisibility ----------" {
        # "Template Separator\n(You can make a copy of, or modify, this frame)"
        n106 = call <vilib>:"Add State(s) to Queue__jki_lib_state_machine.vi"("State(s) in (\"\")"=w256) -> ("States Out"=w255:string)  [unwired: 14 in]
      }
      frame "CV: Previous" {
        # "Template Separator\n(You can make a copy of, or modify, this frame)"
        n107 = property on="Tab Control" class="TabCtl (strict)"(error in=w258) -> (error out=w259:errorcluster, "Value"=w263:enum32{"1", "2", "3", "4", "5", "6", "7"})  [unwired: 1 in, 1 out]
        n108 = Equal To 0?(x=w263) -> (x = 0?=w261:bool)
        n109 = Not(x=w261) -> (.not. x?=w260:bool)
        n110 = property on="Previous Button" class="Bool (strict)"(error in=w259, "Visible"=w260) -> (error out=w257:errorcluster)  [unwired: 1 in, 1 out]
        n111 = call <vilib>:"Add State(s) to Queue__jki_lib_state_machine.vi"("State(s) in (\"\")"=w265) -> ("States Out"=w264:string)  [unwired: 14 in]
      }
      frame "CV: Next" {
        # "Template Separator\n(You can make a copy of, or modify, this frame)"
        n112 = property on="Tab Control" class="TabCtl (strict)"() -> ("Value"=w269:enum32{"1", "2", "3", "4", "5", "6", "7"})  [unwired: 2 in, 2 out]
        n113 = Unbundle By Name(w273) -> ("No of pages"=w267:i32)
        n114 = To Unsigned Byte Integer(number=w269) -> (unsigned 8bit integer=w268:u8)
        n115 = To Unsigned Byte Integer(number=w267) -> (unsigned 8bit integer=w266:u8)
        n116 = Increment(x=w268) -> (x+1=w270:u8)
        n117 = Equal?(x=w266, y=w270) -> (x = y?=w272:bool)
        n118 = Not(x=w272) -> (.not. x?=w271:bool)
        n119 = property on="Next Button" class="Bool (strict)"("Visible"=w271) -> ()  [unwired: 2 in, 2 out]
        n120 = call <vilib>:"Add State(s) to Queue__jki_lib_state_machine.vi"("State(s) in (\"\")"=w276) -> ("States Out"=w275:string)  [unwired: 14 in]
      }
      frame "CV: Done" {
        # "Template Separator\n(You can make a copy of, or modify, this frame)"
        n121 = Unbundle By Name(w283) -> ("No of pages"=w279:i32)
        n122 = property on="Tab Control" class="TabCtl (strict)"() -> ("Value"=w280:enum32{"1", "2", "3", "4", "5", "6", "7"})  [unwired: 2 in, 2 out]
        n123 = To Unsigned Byte Integer(number=w280) -> (unsigned 8bit integer=w281:u8)
        n124 = Increment(x=w281) -> (x+1=w277:u8)
        n125 = To Unsigned Byte Integer(number=w279) -> (unsigned 8bit integer=w278:u8)
        n126 = Equal?(x=w278, y=w277) -> (x = y?=w282:bool)
        n127 = property on="OK Button" class="Bool (strict)"("Visible"=w282) -> ()  [unwired: 2 in, 2 out]
        n128 = call <vilib>:"Add State(s) to Queue__jki_lib_state_machine.vi"("State(s) in (\"\")"=w286) -> ("States Out"=w285:string)  [unwired: 14 in]
      }
      frame "CV: Cancel" {
        # "Template Separator\n(You can make a copy of, or modify, this frame)"
        n129 = call <vilib>:"Add State(s) to Queue__jki_lib_state_machine.vi"("State(s) in (\"\")"=w290) -> ("States Out"=w289:string)  [unwired: 14 in]
      }
      frame "New Category: 1" {
        # "Your code here.\n(You can make a copy of, or modify, this frame)"
        n130 = call <vilib>:"Add State(s) to Queue__jki_lib_state_machine.vi"("State(s) in (\"\")"=w294) -> ("States Out"=w293:string)  [unwired: 14 in]
      }
      frame "New Category: 2" {
        # "Your code here.\n(You can make a copy of, or modify, this frame)"
        n131 = call <vilib>:"Add State(s) to Queue__jki_lib_state_machine.vi"("State(s) in (\"\")"=w298) -> ("States Out"=w297:string)  [unwired: 14 in]
      }
    }
  }
  "Cancel" <- w5
  "error out" <- w1
  n132 = Unbundle By Name(w4) -> ("alarm settings"=→"alarm settings":T1)
